vi "lipo.vi"() -> ()   [LabVIEW 2012]
panel:
  out "Remaining Percentage":dbl
  out "Alarm":bool
  in  "Numeric Control":u32
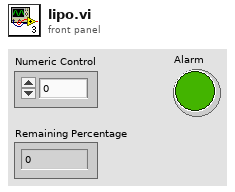
[diagram p1: front panel]
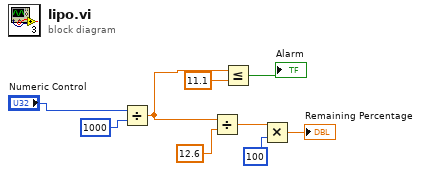
[diagram p0: block diagram]
diagram:
  n1 = Divide(x="Numeric Control", y=1000) -> (x/y=w5:dbl)
  n2 = Divide(x=w5, y=12.6) -> (x/y=w7:dbl)
  n3 = Less Or Equal?(x=w5, y=11.1) -> (x <= y?=→"Alarm":bool)
  n4 = Multiply(x=w7, y=100) -> (x*y=→"Remaining Percentage":dbl)
